vi "set address.destination.vi"(6 "timeout (25000ms)":i32=25000, 8 "error in (no error)":errorcluster, 10 "Target":T1="DDM", 11 "daemon reference in":refnum<k5>) -> (0 "error out":errorcluster, 2 "response":string, 3 "daemon reference out":refnum<k5>, 4 "parameter(s) out":string, 5 "command out":string="set_destination_address")   [LabVIEW 2017]
doc: "<b>Command: </b>\"set_destination_address\"\n\n<b>Description: </b> This command instructs the Daemon to change the DIPC destination address.\n\n<b>Parameters: </b>\n\n 1. Destination Address\n____________________________________________\nDIPC 692 Daemon API 10.0.0.1\nSam Tee - Dyson Technology Ltd\nCopyright (c) 2024, Dyson Technology Ltd"
uses:
  typdef/destination.ctl
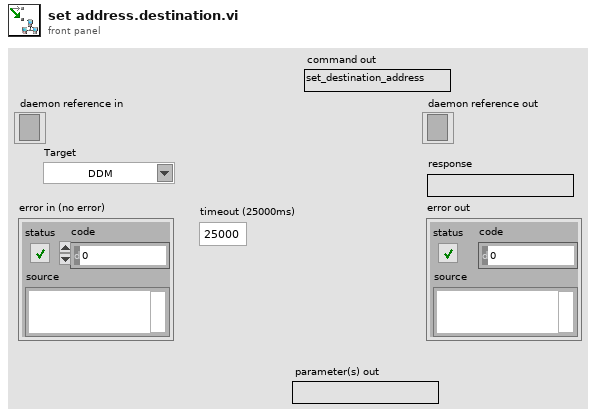
[diagram p1: front panel]
types:
  T1 = typedef "destination.ctl" = string
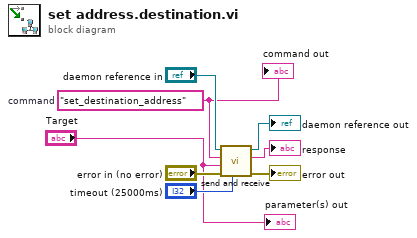
[diagram p0: block diagram]
diagram:
  w6 = "set_destination_address"  # command
  n1 = call "send and receive.vi"("timeout (25000ms)"="timeout (25000ms)", "error in (no error)"="error in (no error)", "data"="Target", "command"=w6, "daemon reference in"="daemon reference in") -> ("error out"=→"error out":errorcluster, "response"=→"response":string, "daemon reference out"=→"daemon reference out":refnum<k5>)  [unwired: 4 in]
  "command out" <- w6
  "parameter(s) out" <- "Target"
